vi "SoundModule.vi"(8 "error out":errorcluster, 10 "Current":dbl(slide) min=0.0 max=1e-09 scale=1e-15..1e-09, 11 "task ID":T1 format="%.0x") -> (0 "error in (no error)":errorcluster, 3 "task ID 2":T1 format="%.0x")   [LabVIEW 2017]
doc: "This VI illustrates how to generate and play sine, square, sawtooth and triangle waveforms. You can change the frequency and type of the waveform generated as it plays continuously."
uses:
  <vilib>/sound2/lvsound2.llb/Sound Output Task ID.ctl
  <vilib>/sound2/lvsound2.llb/Sound Output Set Volume (Single).vi
  <vilib>/sound2/lvsound2.llb/Sound Output Write (DBL Single).vi
  <vilib>/measure/NI_MABase.lvlib
panel:
  in  "Volume 3":dbl(slide)=50.0 scale=0.0..100.0
  out "Generated Sound 3":waveform(dbl)(graph)
  # "out"
  # "in"
  # "Overview: Demonstrates the use of the Sound Functions to generate and play a sine waveform continuously.\nInstructions:\n1. Specify the Device ID.\n2. Run the VI. Waveforms are generated and sent to both the graph and your speakers.\n3. Change the Frequency and Volume of the sound.\n4. Click Stop to stop the VI."
  # "https://forums.ni.com/t5/LabVIEW/Continuous-sound-output-buffer-issue-s/td-p/685140?profile.language=en"
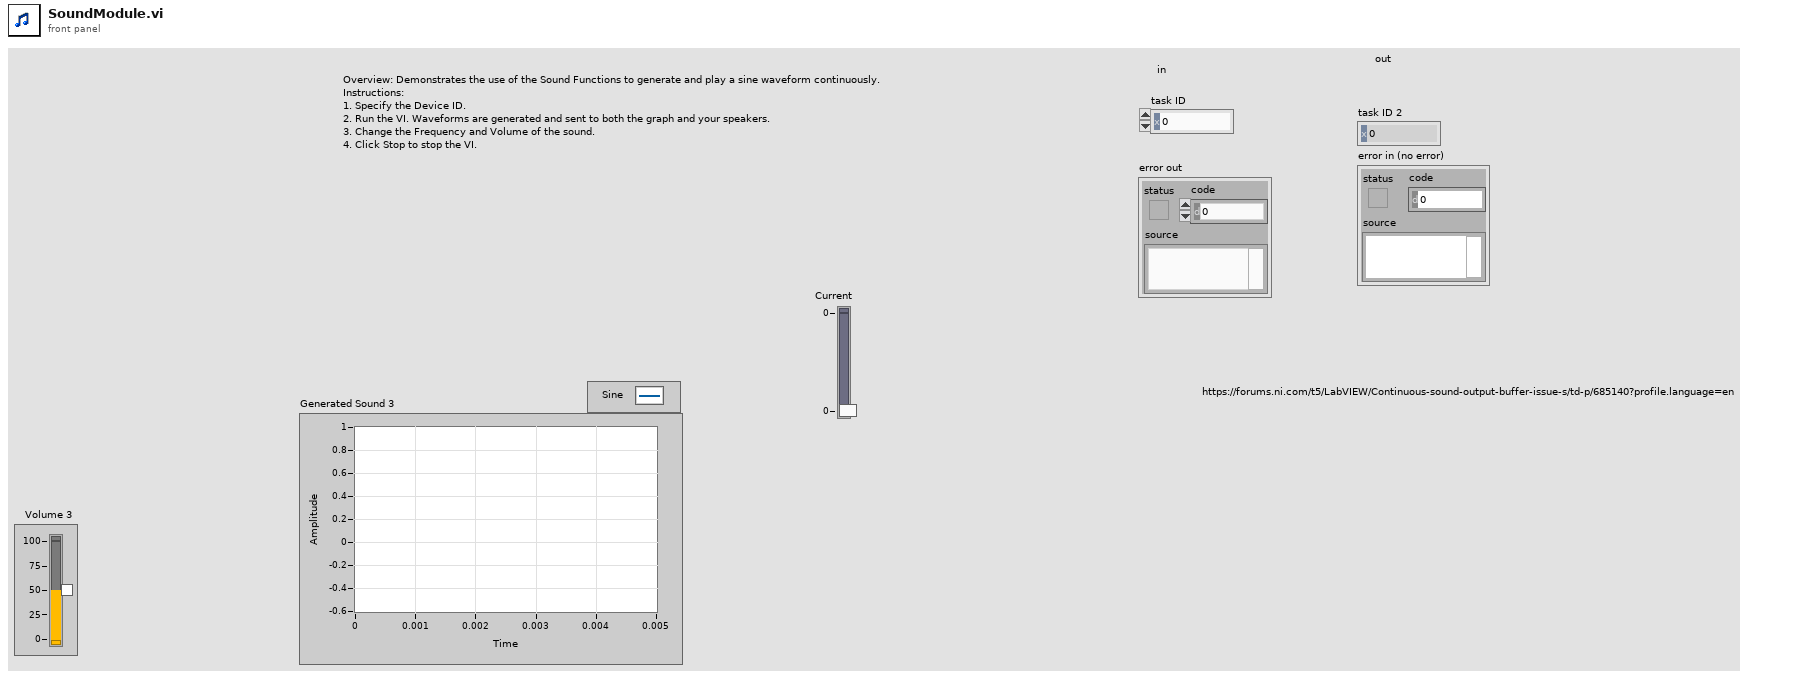
[diagram p1: front panel]
types:
  T1 = typedef "Sound Output Task ID.ctl" = u32
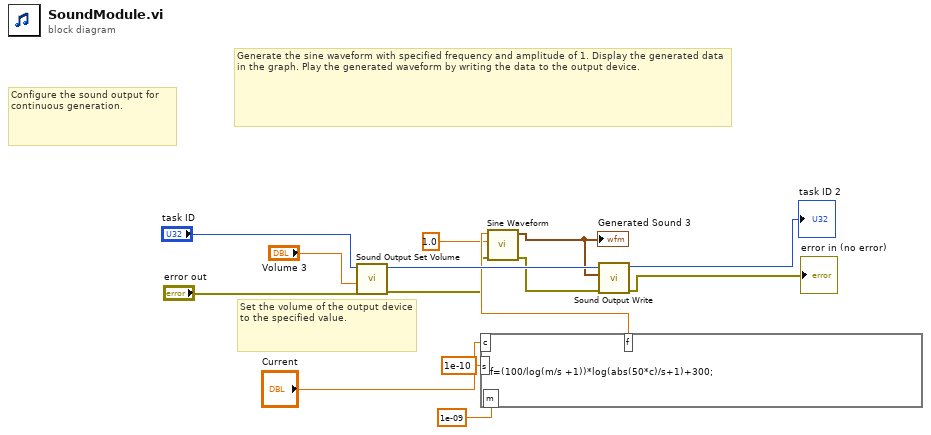
[diagram p0: block diagram]
diagram:
  # "Set the volume of the output device to the specified value."
  # "Generate the sine waveform with specified frequency and amplitude of 1. Display the generated data in the graph. Play the generated waveform by writing the data to the output device."
  # "Configure the sound output for continuous generation."
  n1 = call-poly <vilib>:"Sound Output Set Volume.vi"("error in (no error)"="error out", "volume"="Volume 3", "task ID"="task ID") -> ("error out"=w3:errorcluster, "task ID out"=w14:T1)  [unwired: 7 in]
  n2 = formula code="f=(100/log(m/s +1))*log(abs(50*c)/s+1)+300;"("c"="Current", "s"=1e-10 ("input variable"), "m"=1e-09 ("input variable")) -> ("f"=w4:dbl)
  n3 = call <vilib>:"Sine Waveform.vi"("error in (no error)"=w3, "amplitude"=1.0, "frequency"=w4) -> ("error out"=w2:errorcluster, "signal out"=w5:waveform(dbl))  [unwired: 7 in]
  "Generated Sound 3" <- w5
  n4 = call-poly <vilib>:"Sound Output Write.vi"("error in (no error)"=w2, "data"=w5, "task ID"=w14) -> ("error out"=→"error in (no error)":errorcluster, "task ID out"=→"task ID 2":T1)  [unwired: 7 in]
